vi "Actor Core.vi"(8 "error in":errorcluster, 11 "Alabama Power Remote in":refnum<class "Alabama Power Remote.lvclass">) -> (0 "error out":errorcluster, 3 "Actor out":refnum<class "Actor.lvclass">)   [LabVIEW 2018, in "Alabama Power Remote Actor.lvlib" / "Alabama Power Remote.lvclass"]
doc: "(<B>Filename</B>: Actor Framework.lvlib:Actor.lvclass:Actor Core.vi)\n\nReceives messages to the actor, reacts to them, and initiates any error handling that may shut the actor down.\n\nDescendant classes may override this VI to append parallel tasks for the actor to complete while it handles messages. Overrides use the Call Parent Method node."
uses:
  Alabama Power Remote.lvclass
  C:/Users/Administrator/Desktop/2018LabVIEW EMS/EMS Generic Actor/EMS Generic/EMS Generic.lvclass
  <vilib>/ActorFramework/Actor/Actor.lvclass
  Controls/AP Remote States.ctl
  EMS Generic Actor/EMS Generic/EMS Generic.lvclass/EMS Generic.ctl
  Alabama Power Remote.lvclass/Alabama Power Remote.ctl
  <vilib>/Modbus/master/Create Master Instance (TCP).vi
  Remote Operation Abstract/Remote Operation Abstract.lvclass
  <vilib>/Modbus/master/Modbus Master.lvclass
  EMS Generic Actor/EMS Generic/EMS Generic.lvclass
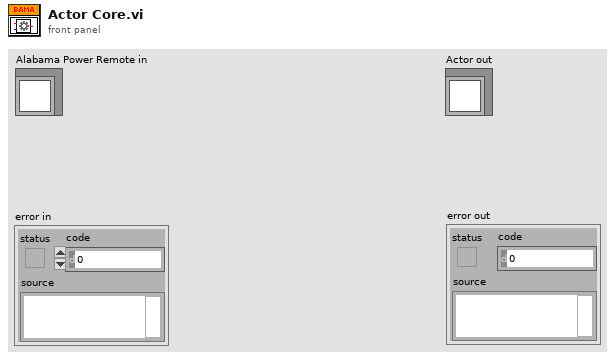
[diagram p1: front panel]
types:
  T1 = typedef "Alabama Power Remote Actor.lvlib/Alabama Power Remote.lvclass/AP Remote States.ctl" = enum16{"Initialize Modbus", "Read Modbus", "Update Points", "Restart", "Shutdown"}
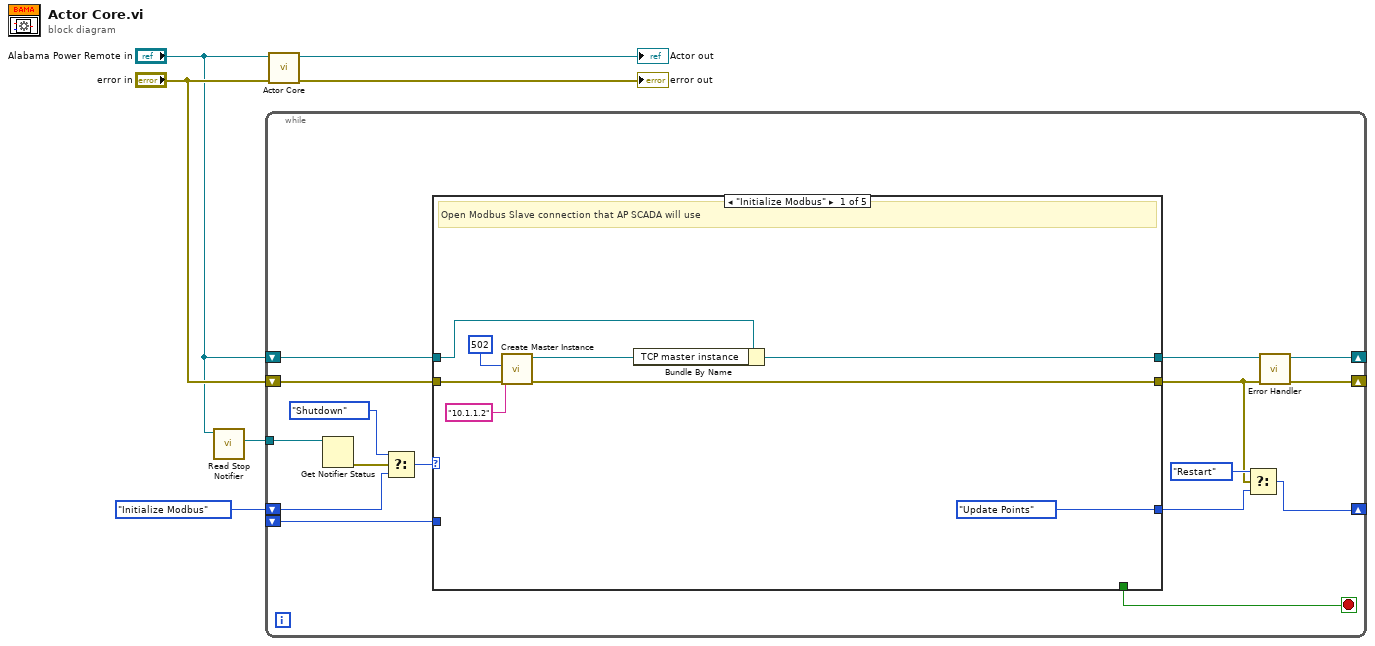
[diagram p0: block diagram]
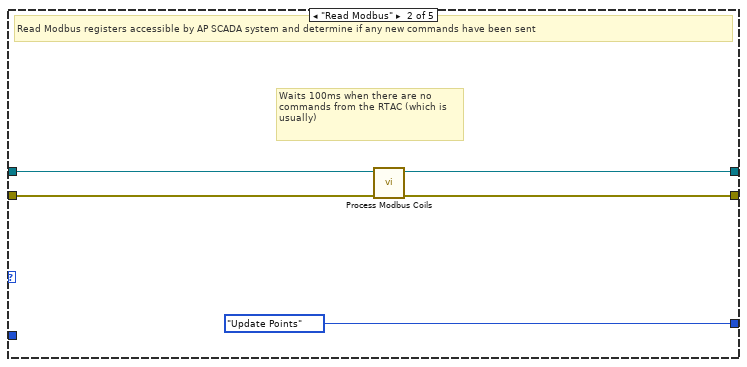
[diagram p2: hidden frame]
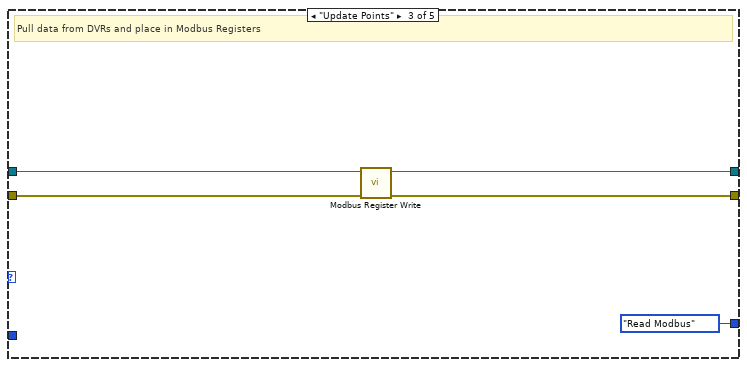
[diagram p3: hidden frame]
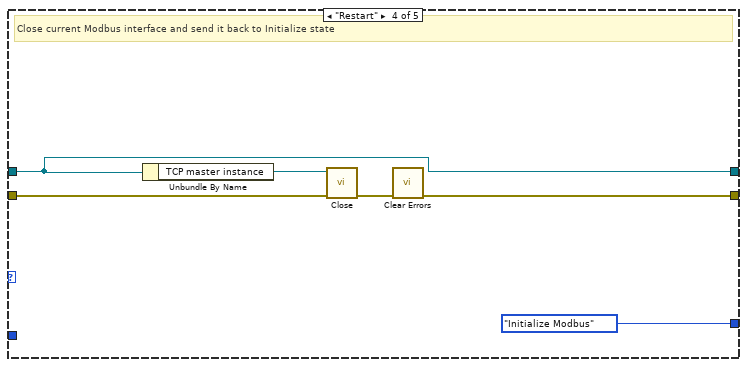
[diagram p4: hidden frame]
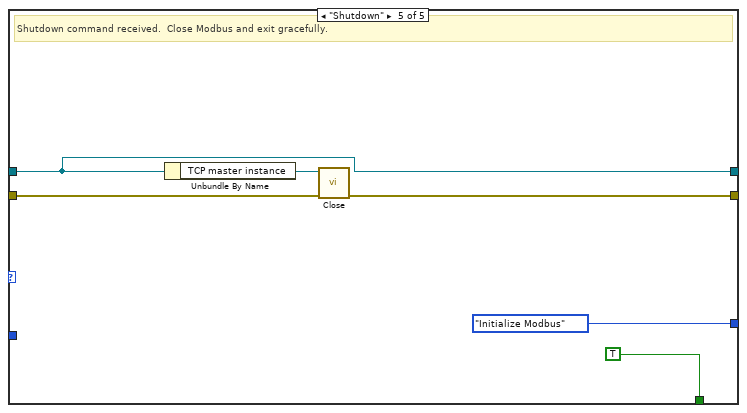
[diagram p5: hidden frame]
diagram:
  w1 = AP_Remote_States."Initialize Modbus"
  n1 = call "Read Stop Notifier.vi"("EMS Generic in"="Alabama Power Remote in") -> ("stop"=w2:refnum<notifier>)  [unwired: 9 in, 1 out]
  n2 = while {
    shift-right: [w17] -> _
    shift-left: w1 -> [w11]
    shift-right: [w8] -> _
    shift-left: "Alabama Power Remote in" -> [w22]
    shift-right: [w15] -> _
    shift-left: "error in" -> [w21]
    tunnel: w2 -> [w14]
    shift-left: w1 -> [w7]
    stop <- w20 stop-if-true
    n3 = Get Notifier Status(notifier=w14) -> (error out=w13:errorcluster)  [unwired: 1 in, 4 out]
    n4 = Select(t=AP_Remote_States."Shutdown", s=w13, f=w11) -> (s? t:f=w10:T1)
    n5 = case shown="\"Initialize Modbus\"" w10 {
      tunnel: [w25 w33 w38 w41 w47] -> w9
      tunnel: [w29 w31 w37 w42 w50] -> w16
      tunnel: w22 -> [w26 w34 w39 w41 w47]
      tunnel: w21 -> [w28 w32 w40 w46 w51]
      tunnel: [AP_Remote_States."Update Points" ("f") AP_Remote_States."Update Points" AP_Remote_States."Read Modbus" ("f") AP_Remote_States."Initialize Modbus" ("f") AP_Remote_States."Initialize Modbus" ("f")] -> w19
      tunnel: [_ _ _ _ TRUE] -> w20
      tunnel: w7 -> [_ _ _ _ _]
      frame "Initialize Modbus" {
        # "Open Modbus Slave connection that AP SCADA will use"
        n6 = call-poly <vilib>:"Create Master Instance.vi"("error in (no error)"=w28, "port (502)"=u16 502, "address"="10.1.1.2") -> ("error out"=w29:errorcluster, "TCP master instance"=w24:refnum<class "Modbus Master.lvclass">)  [unwired: 7 in]
        n7 = Bundle By Name(cluster=w26, "TCP master instance"=w24) -> (w25:refnum<class "Alabama Power Remote.lvclass">)
      }
      frame "Read Modbus" {
        # "Waits 100ms when there are no commands from the RTAC (which is usually)"
        # "Read Modbus registers accessible by AP SCADA system and determine if any new commands have been sent"
        n8 = call "Process Modbus Coils.vi"("error in"=w32, "Alabama Power Remote"=w34) -> ("error out"=w31:errorcluster, "dup Alabama Power Remote"=w33:refnum<class "Alabama Power Remote.lvclass">)  [unwired: 8 in]
      }
      frame "Update Points" {
        # "Pull data from DVRs and place in Modbus Registers"
        n9 = call "Modbus Register Write.vi"("error in"=w40, "Alabama Power Remote in"=w39) -> ("error out"=w37:errorcluster, "Alabama Power Remote out"=w38:refnum<class "Alabama Power Remote.lvclass">)  [unwired: 8 in]
      }
      frame "Restart" {
        # "Close current Modbus interface and send it back to Initialize state"
        n10 = Unbundle By Name(w41) -> ("TCP master instance"=w44:refnum<class "Modbus Master.lvclass">)
        n11 = call-dynamic "Close.vi"("error in (no error)"=w46, "Modbus master in"=w44) -> ("error out"=w43:errorcluster)  [unwired: 9 in]
        n12 = call <vilib>:"Clear Errors.vi"("error in (no error)"=w43) -> ("error out"=w42:errorcluster)  [unwired: 5 in, 1 out]
      }
      frame "Shutdown" {
        # "Shutdown command received.  Close Modbus and exit gracefully."
        n13 = Unbundle By Name(w47) -> ("TCP master instance"=w48:refnum<class "Modbus Master.lvclass">)
        n14 = call-dynamic "Close.vi"("error in (no error)"=w51, "Modbus master in"=w48) -> ("error out"=w50:errorcluster)  [unwired: 9 in]
      }
    }
    n15 = Select(t=AP_Remote_States."Restart", s=w16, f=w19) -> (s? t:f=w17:T1)
    n16 = call-dynamic "Error Handler.vi"("error in"=w16, "Alabama Power Remote in"=w9) -> ("error out"=w15:errorcluster, "Alabama Power Remote out"=w8:refnum<class "Alabama Power Remote.lvclass">)  [unwired: 8 in]
  }
  n17 = call-parent "Actor Core.vi"("error in"="error in", "Actor in"="Alabama Power Remote in") -> ("error out"=→"error out":errorcluster, "Actor out"=→"Actor out":refnum<class "Actor.lvclass">)  [unwired: 8 in]
